vi "patch offset.vi"(1 "VtoPin":dbl[](array[numeric])) -> (0 "VtoPout":dbl[](array[numeric]))   [LabVIEW 2015]
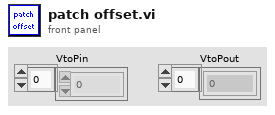
[diagram p1: front panel]
types:
  T1 = cluster{"VC":bool, "CC":bool, "CC_icg (pA/mv)":sgl, "VC_icg (mV/mV)":sgl, "OCG (mV/pA)":sgl, "OVG (mV/mV)":sgl, "Vhold (mV)":sgl, "holdon":bool}
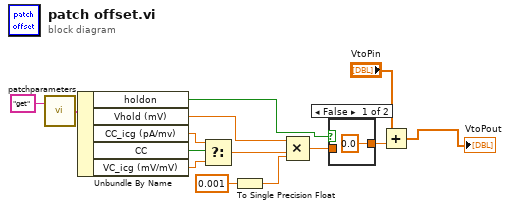
[diagram p0: block diagram]
diagram:
  n1 = call "patchparameters.vi"("command"="get") -> ("Params out"=w10:T1)  [unwired: 1 in]
  n2 = Unbundle By Name(w10) -> ("holdon"=w11:bool, "Vhold (mV)"=w12:sgl, "CC_icg (pA/mv)"=w3:sgl, "CC"=w5:bool, "VC_icg (mV/mV)"=w4:sgl)
  n3 = Select(t=w3, s=w5, f=w4) -> (s? t:f=w2:sgl)
  n4 = To Single Precision Float(number=0.001 ("y")) -> (single precision float=w1:sgl)
  n5 = Compound Arithmetic op=MULTIPLY(w12, w2, w1) -> (w7:sgl)
  n6 = case shown="False" w11 {
    tunnel: w7 -> [_ w16]
    tunnel: [0.0 w16] -> w8
    frame False {
    }
    frame True {
    }
  }
  n7 = Add(x="VtoPin", y=w8) -> (x+y=→"VtoPout":dbl[])
